vi "getfractionalX.vi"(5 "forward":T1=enum."on", 6 "screen [m]":dbl[](array[numeric]), 7 "start index (0)":i32, 9 "position":dbl, 10 "filed of view/pixel":dbl, 11 "Numeric in":i32) -> (2 "index":dbl, 3 "position m":dbl)   [LabVIEW 2011]
uses:
  OnOffTypeDef.ctl
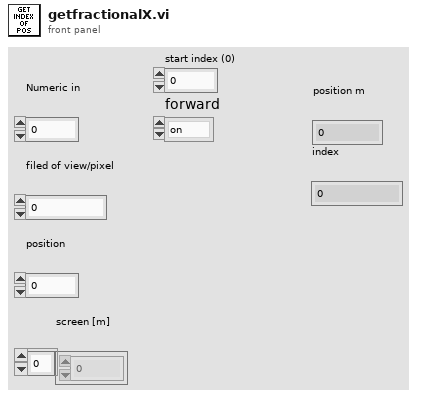
[diagram p1: front panel]
types:
  T1 = typedef "OnOffTypeDef.ctl" = enum16{"off", "on"}
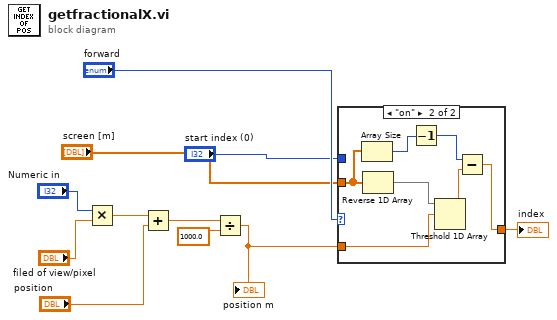
[diagram p0: block diagram]
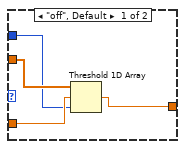
[diagram p2: hidden frame]
diagram:
  n1 = Multiply(x="Numeric in", y="filed of view/pixel") -> (x*y=w7:dbl)
  n2 = Add(x=w7, y="position") -> (x+y=w9:dbl)
  n3 = Divide(x=w9, y=1000.0) -> (x/y=w4:dbl)
  "position m" <- w4
  n4 = case shown="\"on\"" "forward" {
    tunnel: "screen [m]" -> [w15 w20]
    tunnel: w4 -> [w14 w22]
    tunnel: "start index (0)" -> [w13 _]
    tunnel: [w12 w18] -> w2
    frame "off", Default {
      n5 = Threshold 1D Array(1:w13, 2:w14, 3:w15) -> (0:w12:dbl)
    }
    frame "on" {
      n6 = Array Size(array=w20) -> (size(s)=w17:i32)
      n7 = Reverse 1D Array(array=w20) -> (reversed array=w21:dbl[])
      n8 = Decrement(x=w17) -> (x-1=w16:i32)
      n9 = Threshold 1D Array(2:w22, 3:w21) -> (0:w19:dbl)  [unwired: 1 in]
      n10 = Subtract(x=w16, y=w19) -> (x-y=w18:dbl)
    }
  }
  "index" <- w2
